vi "Autonics_1Scan_KAERI_lab2_Daejeon.vi"() -> ()   [LabVIEW 2018]
uses:
  <vilib>/Platform/NI_3dgraph.lvlib
  <vilib>/Utility/file.llb/Write To Spreadsheet File (DBL).vi
  <vilib>/Analysis/Matrix/Datatypes/RealMatrix.ctl
  <vilib>/Analysis/Matrix/NI_Matrix.lvlib
  <resource>/objmgr/daqmx.rc
  <vilib>/Instr/_visa.llb/VISA Configure Serial Port (Instr).vi
  <vilib>/DAQmx/configure/trigger.llb/DAQmx Start Trigger (Digital Edge).vi
  <vilib>/DAQmx/read.llb/DAQmx Read (Analog 2D DBL NChan NSamp).vi
  <vilib>/DAQmx/configure/timing.llb/DAQmx Timing (Sample Clock).vi
  <vilib>/DAQmx/create/channels.llb/DAQmx Create Channel (AI-Voltage-Basic).vi
  <vilib>/Utility/file.llb/Read From Spreadsheet File (DBL).vi
  <vilib>/Analysis/3filter.llb/Filter Passband Type.ctl
  <vilib>/Analysis/NI_AALBase.lvlib
panel:
  in  "Y-min":dbl
  in  "Y-max":dbl
  in  "Trim Data":bool
  in  "X-min":dbl
  in  "X-max":dbl
  out "XY Graph":cluster{"Array Repaired":dbl[], dbl[]}(graph)
  in  "dY":bool
  in  "dX":bool
  in  "Repair Line Y":bool
  in  "Repair Line X":bool
  in  "Line X":dbl
  in  "Line Y":dbl
  in  "Scan Mode":bool
  in  "3D Surface Analysis":refnum<k7>(container)
  in  "Auto Scale ?":bool
  out "Cursor Z":dbl=1.0
  out "Cursor Y":dbl=1.0
  out "Cursor X":dbl=1.0
  in  "Area View":bool
  in  "Save Analysis":bool caption="Save Process"
  in  "Color Max":dbl=1.0 step=0.01
  in  "Color Min":dbl step=0.01
  out "Section View Y":dbl[](graph) caption="Section View"
  in  "ViewMode Analysis":i32(ring) items=["cwViewXYPlane", "cwViewXZPlane", "cwViewYZPlane", "cwViewUserDefined"]
  in  "Plot style Analysis":i32(ring)=5 items=["cwLine"=1, "cwPoint"=2, "cwLinePoint"=3, "cwHiddenLine"=4, "cwSurface"=5, "cwSurfaceLine"=6, "cwSurfaceNormal"=7, "cwContourLine"=8, "cwSurfaceContour"=9]
  in  "Back data Analysis":bool
  in  "Direction":u16(ring) items=["X-dir", "Y-dir"]
  in  "Transpose ?":bool
  in  "filter type":T1
  in  "Filter?":bool
  in  "Order":dbl=2.0
  in  "Low Cutoff Hz":dbl=50.0
  in  "High Cutoff Hz":dbl=300.0
  in  "Sampling Hz":dbl=1000.0
  in  "Open":bool
  in  "Scan Distance":dbl=350.0
  in  "Save Button":bool caption="Save Process"
  in  "ViewMode":i32(ring) items=["cwViewXYPlane", "cwViewXZPlane", "cwViewYZPlane", "cwViewUserDefined"]
  in  "Back data":bool
  in  "Data Type":u16(ring) items=["Normal", "dX", "dY"]
  in  "Sampling Rate(Hz)":dbl=15000.0
  in  "Samples per Channels":i32=1000
  in  "Min Volts":dbl=-10.0 format="%0.2f"
  in  "Max Volts":dbl=10.0 format="%0.2f"
  in  "Channels":tag="Dev3/ai0:63"
  in  "Scan Step (mm)":dbl=1.0
  in  "Scan":bool
  in  "Plot style":i32(ring)=5 items=["cwLine"=1, "cwPoint"=2, "cwLinePoint"=3, "cwHiddenLine"=4, "cwSurface"=5, "cwSurfaceLine"=6, "cwSurfaceNormal"=7, "cwContourLine"=8, "cwSurfaceContour"=9]
  in  "3D Surface":refnum<k7>(container)
  in  "Flow control":u16(ring) items=["None", "XON/XOFF", "RTS/CTS", "XON/XOFF & RTS/CTS", "DTR/DSR", "XON/XOFF & DTR/DSR"]
  in  "Stop bits":u16(ring)=10 items=["1.0"=10, "1.5"=15, "2.0"=20]
  in  "Parity":dbl
  in  "Data bits":u16=8 min=5 max=8 step=1
  in  "Baud Rate":u32=57600
  in  "COM Port":refnum<visa-resource-name>="COM3"
  in  "Speed":dbl=10.0
  out "Current  Position (mm)":dbl format="%#_4g"
  in  "Move Distance (mm)":dbl=20.0
  in  "Stop Scan":bool
  in  "Stop":bool
  in  "Home":bool
  in  "Right":bool
  in  "Left":bool
  # "SCANNER CONTROL"
  # "BOBBIN-TYPE MAGNETIC CAMERA"
  # "CHANNELS"
  # "COM Setting"
  # "TIMING"
  # "DATA ANALYSIS"
  # "Filters"
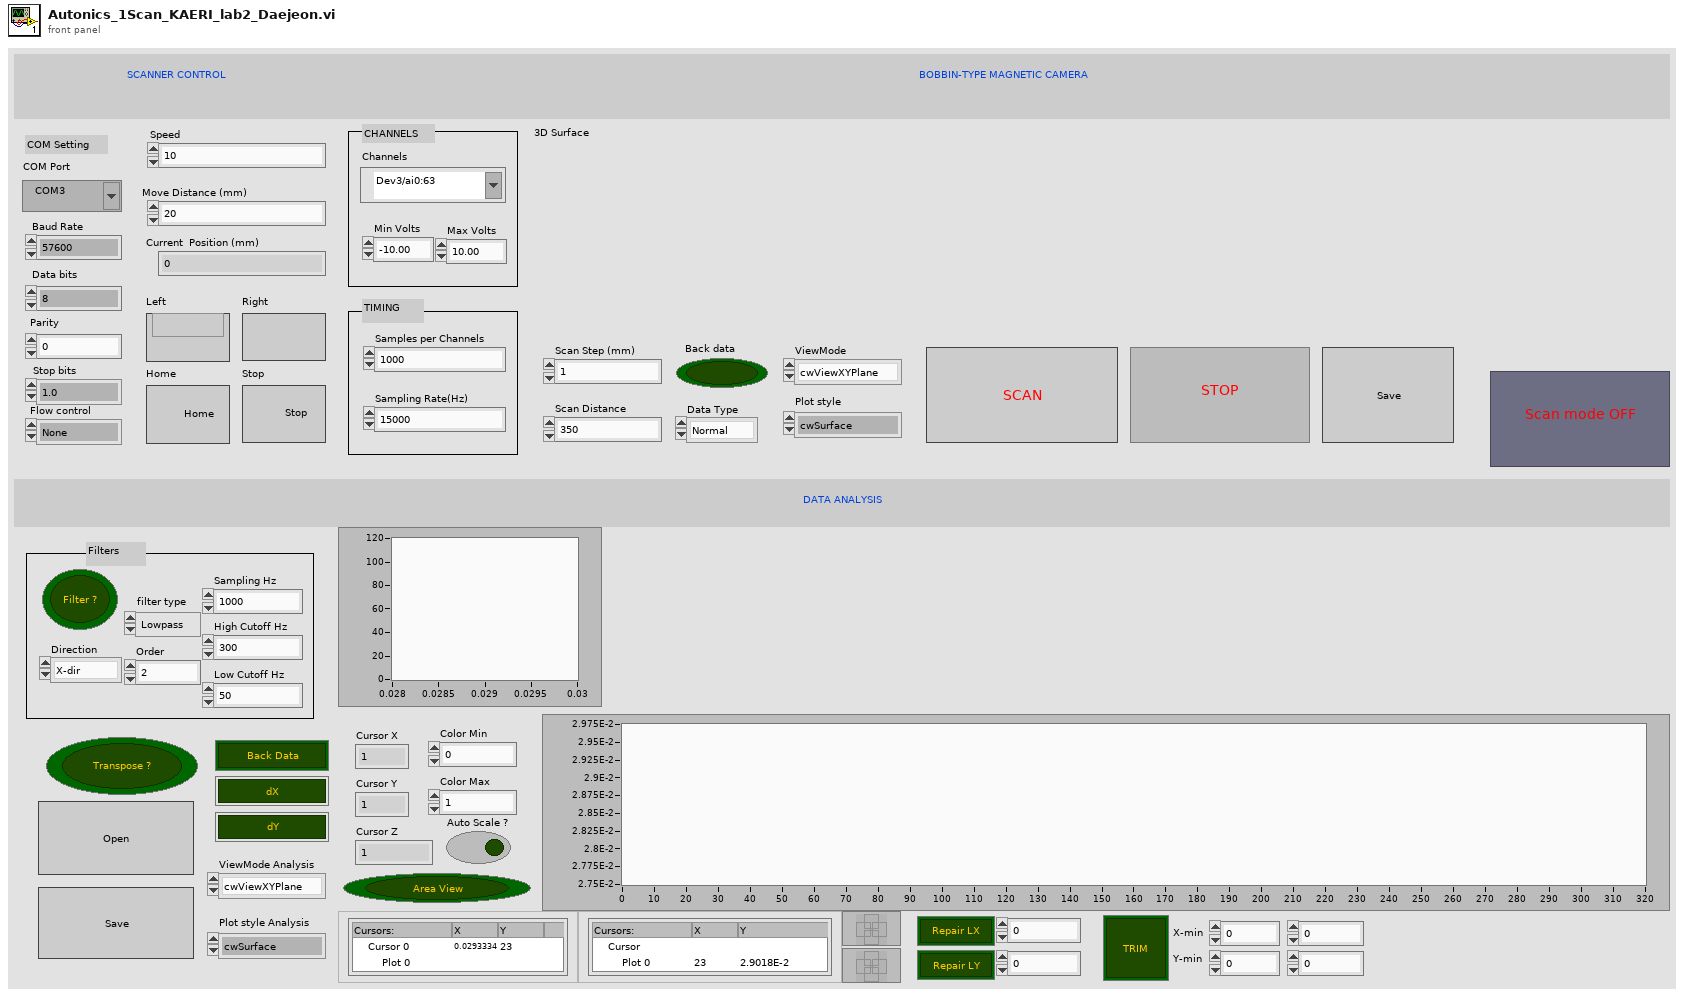
[diagram p1: front panel]
types:
  T1 = typedef "NI_AALBase.lvlib/Filter Passband Type.ctl" = enum32{"Lowpass", "Highpass", "Bandpass", "Bandstop"}
  T2 = typedef "NI_Matrix.lvlib/RealMatrix.ctl" = dbl[][]
  T3 = enum32{"Invalid", "Standard", "Closed", "Hidden", "Minimized", "Maximized"}
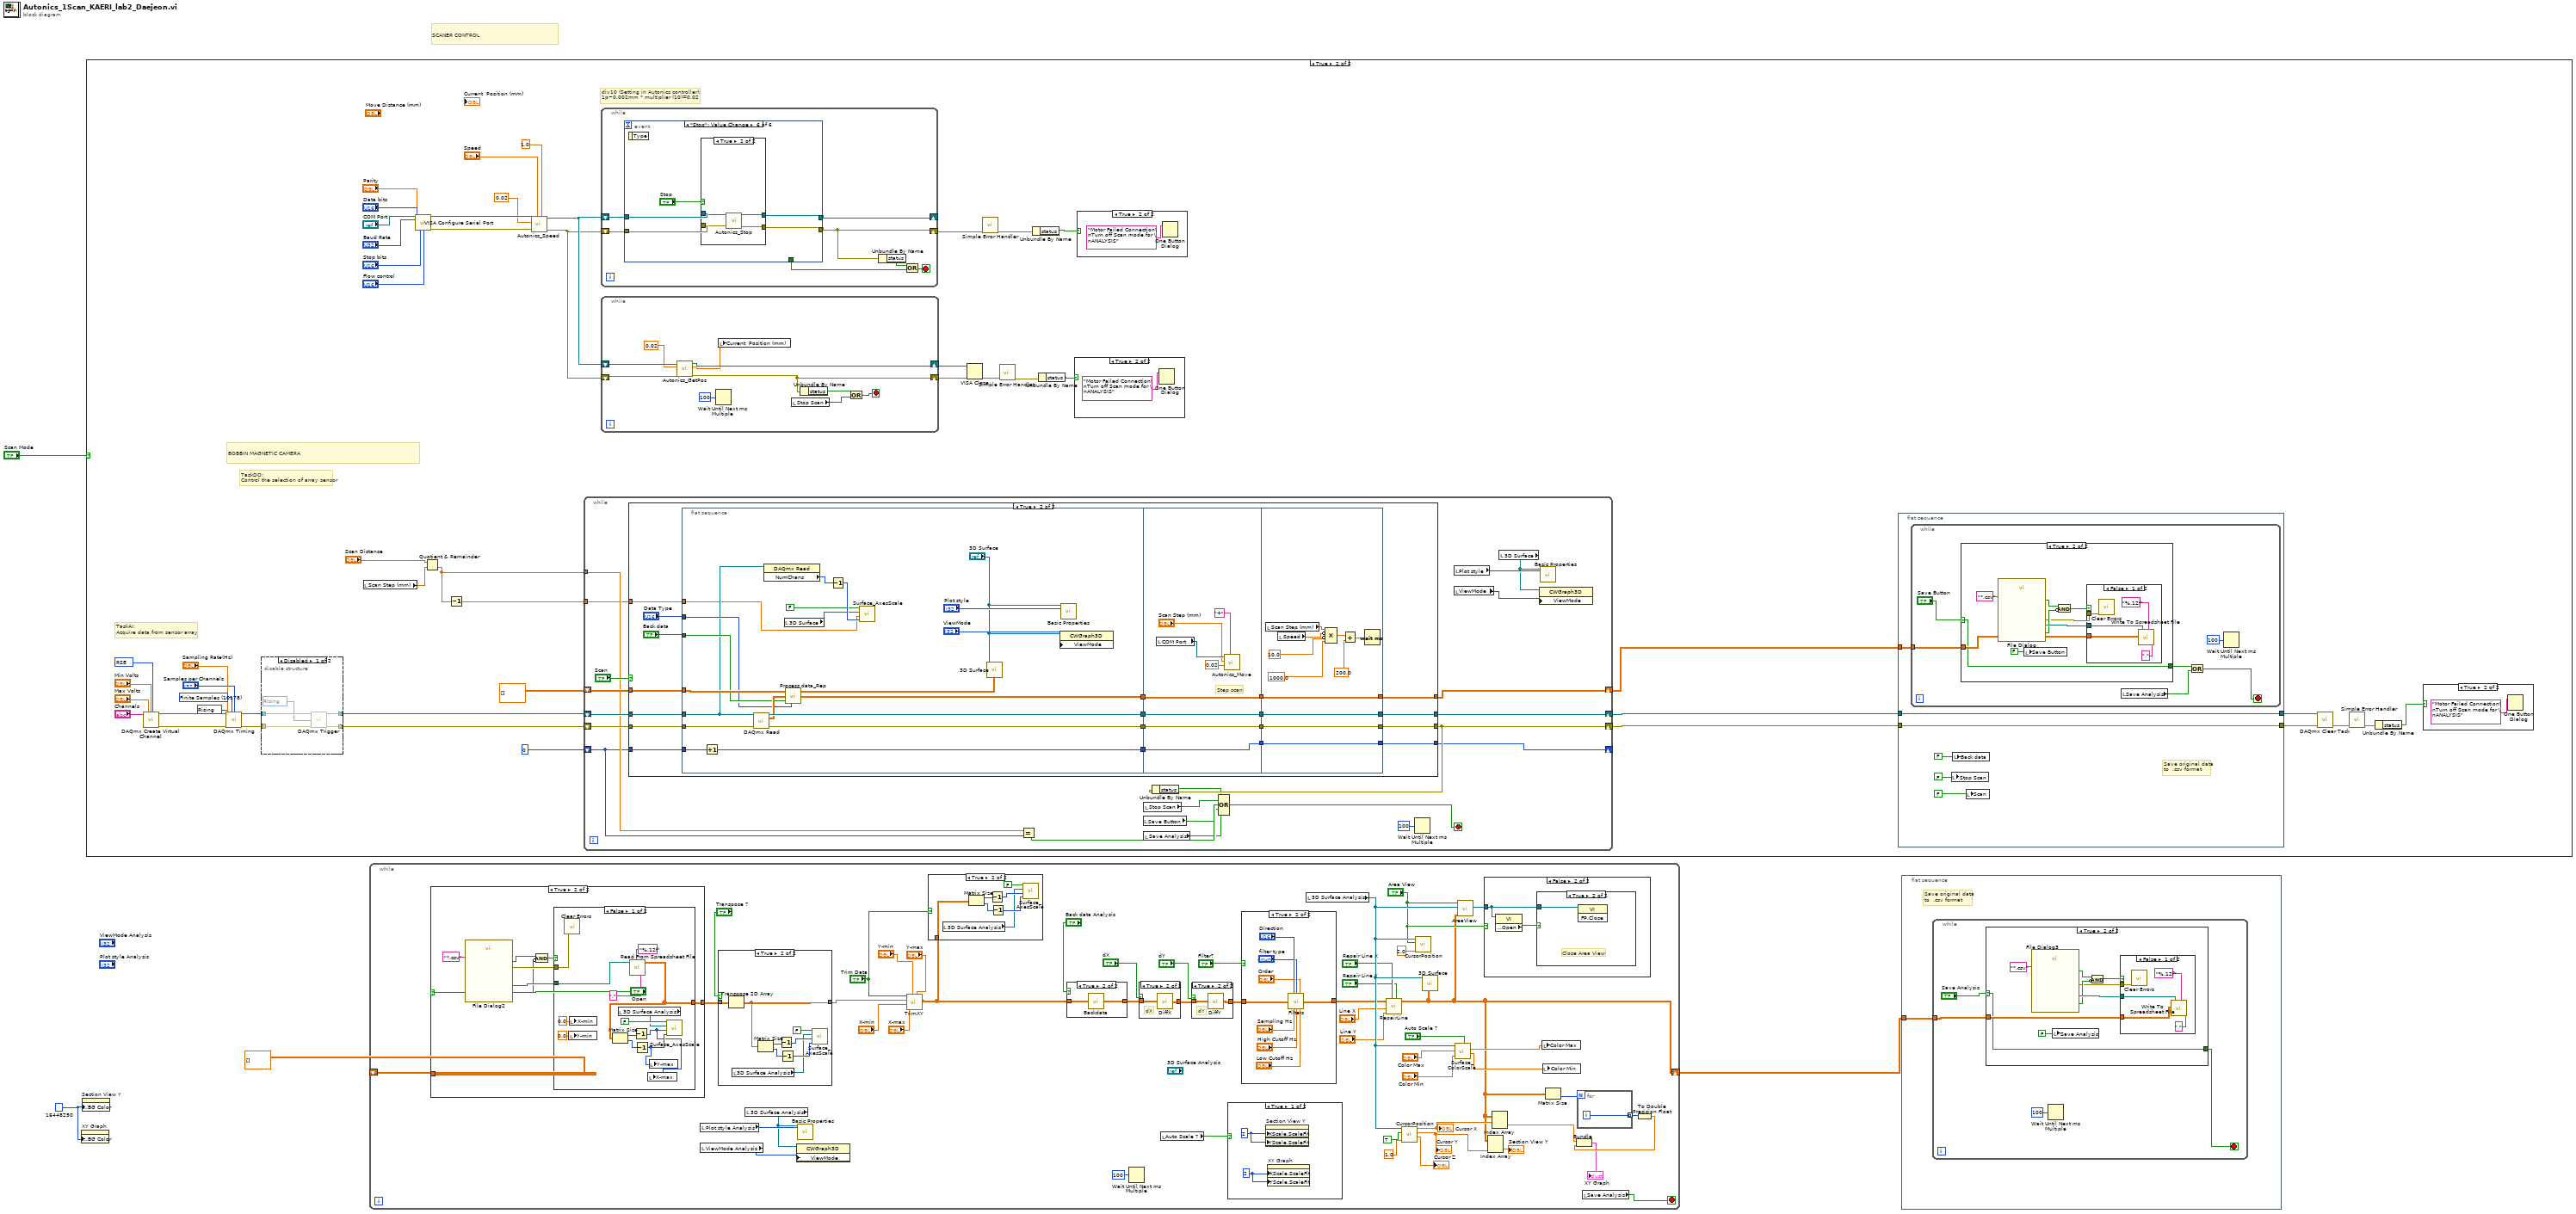
[diagram p0: block diagram]
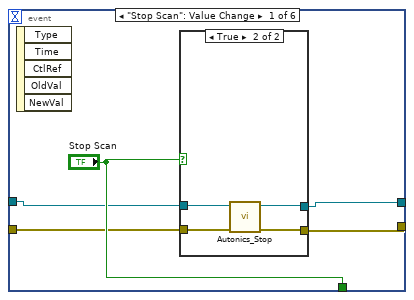
[diagram p6: hidden frame]
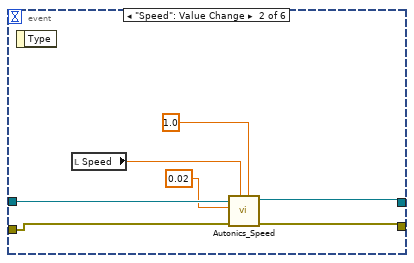
[diagram p8: hidden frame]
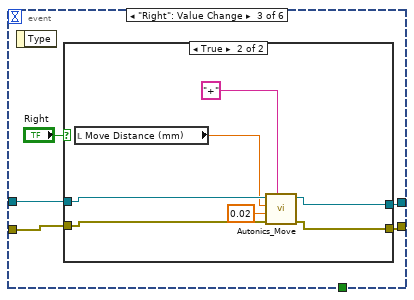
[diagram p9: hidden frame]
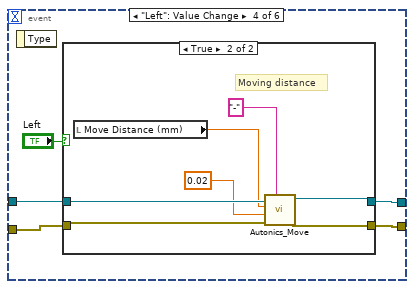
[diagram p11: hidden frame]
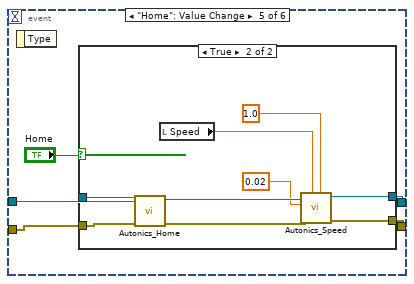
[diagram p13: hidden frame]
diagram:
  w1 = u32 16448250
  # "SCANER CONTROL"
  n1 = property on="XY Graph" class="XYGraph (strict)"("Plot Area:Colors:BG Color"=w1) -> ()  [unwired: 2 in, 2 out]
  n2 = property on="Section View Y" class="WFGraph (strict)"("Plot Area:Colors:BG Color"=w1) -> ()  [unwired: 2 in, 2 out]
  n3 = case shown="True" "Scan Mode" {
    frame False {
    }
    frame True {
      w36 = 10280 items=["Rising"=10280, "Falling"=10171] ("active edge")
      w45 = 10083 items=["default"=-1, "RSE"=10083, "NRSE"=10078, "Differential"=10106, "Pseudodifferential"=12529] ("input terminal configuration")
      w46 = 10178 items=["Finite Samples"=10178, "Continuous Samples"=10123, "Hardware Timed Single Point"=12522] ("sample mode")
      # "div10 (Setting in Autonics controller):\n1p~0.002mm * multiplier (10)=0.02"
      # "TaskAI:\nAcquire data from sensor array"
      # "TaskDO: \nControl the selection of array sensor"
      # "BOBBIN MAGNETIC CAMERA"
      n4 = call-poly <vilib>:"DAQmx Create Virtual Channel.vi"("maximum value"="Max Volts", "minimum value"="Min Volts", "input terminal configuration"=w45, "physical channels"="Channels") -> ("task out"=w53:refnum<k21>, "error out"=w52:errorcluster)  [unwired: 10 in]
      n5 = call-poly <vilib>:"DAQmx Timing.vi"("task/channels in"=w53, "sample mode"=w46, "samples per channel"="Samples per Channels", "rate"="Sampling Rate(Hz)", "active edge"=w36, "error in"=w52) -> ("task out"=w35:refnum<k21>, "error out"=w34:errorcluster)  [unwired: 8 in]
      n6 = disable-structure shown="Disabled" {
        disable-tunnel: w35 -> [w152 w154]
        disable-tunnel: [w151 w154] -> w30
        disable-tunnel: w34 -> [w150 w153]
        disable-tunnel: [w149 w153] -> w33
        frame Disabled {
          w148 = 10280 items=["Rising"=10280, "Falling"=10171] ("edge")
          n7 = call-poly <vilib>:"DAQmx Trigger.vi"("task/channels in"=w152, "edge"=w148, "error in"=w150) -> ("task out"=w151:refnum<k21>, "source"=w147:tag, "error out"=w149:errorcluster)  [unwired: 10 in]
        }
        frame Enabled {
        }
      }
      n8 = local read "Scan Step (mm)"() -> (w44:dbl)
      n9 = call-poly "VISA Configure Serial Port"("VISA resource name"="COM Port", "baud rate (9600)"="Baud Rate", "data bits (8)"="Data bits", "parity (0:none)"="Parity", "stop bits (10: 1 bit)"="Stop bits", "flow control (0:none)"="Flow control") -> ("VISA resource name out"=w16:refnum<visa-resource-name>, "error out"=w15:errorcluster)  [unwired: 8 in]
      n10 = Quotient & Remainder(x="Scan Distance", y=w44) -> (floor(x/y)=w32:dbl)  [unwired: 1 out]
      n11 = Decrement(x=w32) -> (x-1=w28:dbl)
      n12 = call "Autonics_Speed.vi"("Multiplier"=1.0, "Speed (mm/s)"="Speed", "error in (no error)"=w15, "Travel per  Pulse"=0.02, "VISA resource name"=w16) -> ("error out"=w18:errorcluster, "VISA resource name out"=w19:refnum<visa-resource-name>)  [unwired: 5 in]
      n13 = while {
        shift-right: [w185] -> w29
        shift-left: T2 [] ("Output (Matrix)") -> [w201]
        shift-right: [w199] -> w40
        shift-left: w30 -> [w200]
        shift-right: [w195] -> w38
        shift-left: w33 -> [w202]
        shift-right: [w193] -> _
        shift-left: 0 -> [w191]
        tunnel: w32 -> [w192]
        tunnel: w28 -> [w184]
        stop <- w198 stop-if-true
        n14 = case shown="True" "Scan" {
          tunnel: w200 -> [w205 w225]
          tunnel: w202 -> [w204 w224]
          tunnel: w201 -> [w203 w223]
          tunnel: [w205 w219] -> w199
          tunnel: [w204 w218] -> w195
          tunnel: [w203 w208] -> w185
          tunnel: [w206 w215] -> w193
          tunnel: w191 -> [w206 w213]
          tunnel: w184 -> [_ w207]
          frame False {
          }
          frame True {
            n15 = flat-sequence {
              tunnel: [w244] -> w222
              tunnel: [w235] -> w221
              tunnel: [w243] -> w220
              tunnel: [w234] -> w214
              tunnel: w225 -> [w227]
              tunnel: w224 -> [w245]
              tunnel: w223 -> [w239]
              tunnel: "Back data" -> [w237]
              tunnel: "Data Type" -> [w236]
              tunnel: w213 -> [w233]
              tunnel: w207 -> [w226]
              tunnel: w222 -> [w253]
              tunnel: w221 -> [w252]
              tunnel: w220 -> [w251]
              tunnel: w214 -> [w250]
              tunnel: [w253] -> w212
              tunnel: [w252] -> w211
              tunnel: [w251] -> w210
              tunnel: [w250] -> w209
              tunnel: [w261] -> w215
              tunnel: [w262] -> w218
              tunnel: [w263] -> w208
              tunnel: [w264] -> w219
              tunnel: w212 -> [w264]
              tunnel: w211 -> [w263]
              tunnel: w210 -> [w262]
              tunnel: w209 -> [w261]
              frame #0 {
                n16 = Increment(x=w233) -> (x+1=w234:i32)
                n17 = call-poly <vilib>:"DAQmx Read.vi"("task/channels in"=w227, "error in"=w245) -> ("task out"=w244:refnum<k21>, "data"=w238:dbl[][], "error out"=w243:errorcluster)  [unwired: 11 in]
                n18 = property class="DAQmx Read"(reference=w227) -> ("NumChans"=w230:u32)  [unwired: 1 in, 2 out]
                n19 = local read "3D Surface"() -> (w229:refnum<k7>)
                n20 = call "Process data_Rep.vi"("Initial Matrix"=w239, "Input Matrix"=w238, "Back Data"=w237, "Data Type"=w236) -> ("Process Output (Matrix)"=w232:T2, "Output (Matrix)"=w235:T2)  [unwired: 2 in]
                n21 = Decrement(x=w230) -> (x-1=w231:u32)
                n22 = call "Surface_AxesScale.vi"("Y-axis Max"=w231, "X-axis max"=w226, "3D Surface"=w229, "Auto Scale"=FALSE) -> ()  [unwired: 8 in]
                n23 = call <vilib>:"3D Surface.vi"("z matrix"=w232, "3D graph"="3D Surface") -> ()  [unwired: 8 in, 2 out]
                n24 = property class="CWGraph3D"(reference="3D Surface", "ViewMode"="ViewMode") -> ()  [unwired: 1 in, 2 out]
                n25 = call <vilib>:"Basic Properties.vi"("3D graph"="3D Surface", "plot style"="Plot style") -> ()  [unwired: 12 in, 2 out]
              }
              frame #1 {
                # "Step scan"
                n26 = local read "COM Port"() -> (w249:refnum<visa-resource-name>)
                n27 = call "Autonics_Move.vi"("Direction (+)"="+", "Travel per Pulse (mm)"=0.02, "Move Distance (mm)"="Scan Step (mm)", "VISA resource name"=w249) -> ()  [unwired: 6 in, 2 out]
              }
              frame #2 {
                n28 = local read "Scan Step (mm)"() -> (w256:dbl)
                n29 = local read "Speed"() -> (w257:dbl)
                n30 = Compound Arithmetic op=MULTIPLY(w256, invert w257, invert 10.0 ("value"), 1000.0 ("value")) -> (w258:dbl)
                n31 = Add(x=w258, y=200.0) -> (x+y=w260:dbl)
                n32 = Wait (ms)(milliseconds to wait=w260) -> ()  [unwired: 1 out]
              }
            }
          }
        }
        n33 = Equal?(x=w192, y=w191) -> (x = y?=w190:bool)
        n34 = local read "Save Button"() -> (w183:bool)
        n35 = local read "Stop Scan"() -> (w196:bool)
        n36 = local read "Save Analysis"() -> (w182:bool)
        n37 = Unbundle By Name(w195) -> ("status"=w194:bool)
        n38 = Compound Arithmetic op=OR(w194, w196, w190, w183, w182) -> (w198:bool)
        n39 = Wait Until Next ms Multiple(millisecond multiple=u32 100) -> ()  [unwired: 1 out]
        n40 = local read "Plot style"() -> (w188:i32)
        n41 = local read "ViewMode"() -> (w187:i32)
        n42 = local read "3D Surface"() -> (w186:refnum<k7>)
        n43 = property class="CWGraph3D"(reference=w186, "ViewMode"=w187) -> ()  [unwired: 1 in, 2 out]
        n44 = call <vilib>:"Basic Properties.vi"("3D graph"=w186, "plot style"=w188) -> ()  [unwired: 12 in, 2 out]
      }
      n45 = while {
        shift-right: [w73] -> _
        shift-left: w19 -> [w72]
        shift-right: [w69] -> w10
        shift-left: w18 -> [w71]
        stop <- w68 stop-if-true
        n46 = event shown="[5] \"Stop\": Value Change" {
          selector: _ -> [_ _ _ _ _ _]
          dyn-events: _ -> [_ _ _ _ _ _]
          timeout: _ -> [_ _ _ _ _ _]
          tunnel: w72 -> [w77 w91 w94 w108 w124 w138]
          tunnel: w71 -> [w76 w90 w93 w107 w123 w137]
          tunnel: [w75 w87 w96 w110 w121 w140] -> w73
          tunnel: [w74 w88 w95 w109 w120 w139] -> w69
          tunnel: ["Stop Scan" _ _ _ _ _] -> w67
          event "Stop Scan": Value Change {
            n47 = event-data() -> ()  [unwired: 1 in, 5 out]
            n48 = case shown="True" "Stop Scan" {
              tunnel: [w80 w83] -> w75
              tunnel: [w79 w84] -> w74
              tunnel: w77 -> [w80 w82]
              tunnel: w76 -> [w79 w81]
              frame False {
              }
              frame True {
                n49 = call "Autonics_Stop.vi"("error in (no error)"=w81, "VISA resource name"=w82) -> ("error out"=w84:errorcluster, "VISA resource name out"=w83:refnum<visa-resource-name>)  [unwired: 8 in]
              }
            }
          }
          event "Speed": Value Change {
            n50 = event-data() -> ()  [unwired: 1 in, 1 out]
            n51 = local read "Speed"() -> (w89:dbl)
            n52 = call "Autonics_Speed.vi"("Multiplier"=1.0, "Speed (mm/s)"=w89, "error in (no error)"=w90, "Travel per  Pulse"=0.02, "VISA resource name"=w91) -> ("error out"=w88:errorcluster, "VISA resource name out"=w87:refnum<visa-resource-name>)  [unwired: 5 in]
          }
          event "Right": Value Change {
            n53 = event-data() -> ()  [unwired: 1 in, 1 out]
            n54 = case shown="True" "Right" {
              tunnel: [w97 w103] -> w96
              tunnel: [w98 w102] -> w95
              tunnel: w94 -> [w97 w105]
              tunnel: w93 -> [w98 w104]
              frame False {
              }
              frame True {
                n55 = local read "Move Distance (mm)"() -> (w101:dbl)
                n56 = call "Autonics_Move.vi"("Direction (+)"="+", "error in (no error)"=w104, "Travel per Pulse (mm)"=0.02, "Move Distance (mm)"=w101, "VISA resource name"=w105) -> ("error out"=w102:errorcluster, "VISA resource name out"=w103:refnum<visa-resource-name>)  [unwired: 5 in]
              }
            }
          }
          event "Left": Value Change {
            n57 = event-data() -> ()  [unwired: 1 in, 1 out]
            n58 = case shown="True" "Left" {
              tunnel: [w112 w117] -> w110
              tunnel: [w111 w116] -> w109
              tunnel: w108 -> [w112 w119]
              tunnel: w107 -> [w111 w118]
              frame False {
              }
              frame True {
                # "Moving distance"
                n59 = local read "Move Distance (mm)"() -> (w114:dbl)
                n60 = call "Autonics_Move.vi"("Direction (+)"="-", "error in (no error)"=w118, "Travel per Pulse (mm)"=0.02, "Move Distance (mm)"=w114, "VISA resource name"=w119) -> ("error out"=w116:errorcluster, "VISA resource name out"=w117:refnum<visa-resource-name>)  [unwired: 5 in]
              }
            }
          }
          event "Home": Value Change {
            n61 = event-data() -> ()  [unwired: 1 in, 1 out]
            n62 = case shown="True" "Home" {
              tunnel: [w126 w130] -> w121
              tunnel: [w125 w129] -> w120
              tunnel: w124 -> [w126 w135]
              tunnel: w123 -> [w125 w134]
              frame False {
              }
              frame True {
                n63 = call "Autonics_Home.vi"("error in (no error)"=w134, "VISA resource name"=w135) -> ("error out"=w131:errorcluster, "VISA resource name out"=w132:refnum<visa-resource-name>)  [unwired: 8 in]
                n64 = local read "Speed"() -> (w133:dbl)
                n65 = call "Autonics_Speed.vi"("Multiplier"=1.0, "Speed (mm/s)"=w133, "error in (no error)"=w131, "Travel per  Pulse"=0.02, "VISA resource name"=w132) -> ("error out"=w129:errorcluster, "VISA resource name out"=w130:refnum<visa-resource-name>)  [unwired: 5 in]
              }
            }
          }
          event "Stop": Value Change {
            n66 = event-data() -> ()  [unwired: 1 in, 1 out]
            n67 = case shown="True" "Stop" {
              tunnel: [w142 w143] -> w140
              tunnel: [w141 w146] -> w139
              tunnel: w138 -> [w142 w145]
              tunnel: w137 -> [w141 w144]
              frame False {
              }
              frame True {
                n68 = call "Autonics_Stop.vi"("error in (no error)"=w144, "VISA resource name"=w145) -> ("error out"=w146:errorcluster, "VISA resource name out"=w143:refnum<visa-resource-name>)  [unwired: 8 in]
              }
            }
          }
        }
        n69 = Unbundle By Name(w69) -> ("status"=w70:bool)
        n70 = Compound Arithmetic op=OR(w70, w67) -> (w68:bool)
      }
      n71 = while {
        shift-right: [w61] -> w21
        shift-left: w19 -> [w63]
        shift-right: [w60] -> w20
        shift-left: w18 -> [w62]
        stop <- w64 stop-if-true
        n72 = call "Autonics_GetPos.vi"("error in (no error)"=w62, "Travel per Pulse (mm)"=0.02, "VISA resource name"=w63) -> ("error out"=w60:errorcluster, "Current  Position (mm)"=w59:dbl, "VISA resource name out"=w61:refnum<visa-resource-name>)  [unwired: 6 in]
        n73 = Wait Until Next ms Multiple(millisecond multiple=u32 100) -> ()  [unwired: 1 out]
        n74 = local write "Current  Position (mm)"(w59) -> ()
        n75 = local read "Stop Scan"() -> (w65:bool)
        n76 = Unbundle By Name(w60) -> ("status"=w57:bool)
        n77 = Compound Arithmetic op=OR(w57, w65) -> (w64:bool)
      }
      n78 = VISA Close(VISA resource name=w21, error in (no error)=w20) -> (error out=w8:errorcluster)
      n79 = call <vilib>:"Simple Error Handler.vi"("error in (no error)"=w10) -> ("error out"=w9:errorcluster)  [unwired: 4 in, 4 out]
      n80 = call <vilib>:"Simple Error Handler.vi"("error in (no error)"=w8) -> ("error out"=w7:errorcluster)  [unwired: 4 in, 4 out]
      n81 = Unbundle By Name(w9) -> ("status"=w12:bool)
      n82 = Unbundle By Name(w7) -> ("status"=w11:bool)
      n83 = case shown="True" w11 {
        frame False {
        }
        frame True {
          n84 = One Button Dialog(message="Motor Failed Connection\nTurn off Scan mode for \nANALYSIS") -> ()  [unwired: 1 in, 1 out]
        }
      }
      n85 = case shown="True" w12 {
        frame False {
        }
        frame True {
          n86 = One Button Dialog(message="Motor Failed Connection\nTurn off Scan mode for \nANALYSIS") -> ()  [unwired: 1 in, 1 out]
        }
      }
      n87 = flat-sequence {
        tunnel: w40 -> [w160]
        tunnel: [w160] -> w39
        tunnel: w38 -> [w159]
        tunnel: [w159] -> w37
        tunnel: w29 -> [w155]
        frame #0 {
          # "Save original data\nto  .csv format"
          n88 = while {
            tunnel: w155 -> [w166]
            stop <- w161 stop-if-true
            n89 = case shown="True" "Save Button" {
              selector: "Save Button" -> [w167 w169]
              tunnel: w166 -> [_ w176]
              tunnel: [w167 w169] -> w163
              frame False {
              }
              frame True {
                n90 = call "File Dialog"("pattern (all files)"="*.csv") -> ("selected path"=w174:path, "exists"=w172:bool, "cancelled"=w173:bool, "error out"=w170:errorcluster)  [unwired: 11 in]
                n91 = local write "Save Button"(FALSE ("Save Button")) -> ()
                n92 = Compound Arithmetic op=AND(w173, invert w172) -> (w171:bool)
                n93 = case shown="False" w171 {
                  tunnel: w176 -> [w181 _]
                  tunnel: w174 -> [w179 _]
                  tunnel: w170 -> [w177 _]
                  frame False {
                    n94 = call <vilib>:"Clear Errors.vi"("error in (no error)"=w177) -> ()  [unwired: 5 in, 2 out]
                    n95 = call-poly <vilib>:"Write To Spreadsheet File.vi"("delimiter (\\t)"="," ("delimiter (\\t)"), "format (%.3f)"="%.12f", "2D data"=w181, "file path (dialog if empty)"=w179) -> ()  [unwired: 4 in, 1 out]
                  }
                  frame True {
                  }
                }
              }
            }
            n96 = local read "Save Analysis"() -> (w162:bool)
            n97 = Compound Arithmetic op=OR(w163, w162) -> (w161:bool)
            n98 = Wait Until Next ms Multiple(millisecond multiple=u32 100) -> ()  [unwired: 1 out]
          }
          n99 = local write "Stop Scan"(FALSE ("Exit")) -> ()
          n100 = local write "Back data"(FALSE ("Back data")) -> ()
          n101 = local write "Scan"(FALSE ("Scan")) -> ()
        }
      }
      n102 = call <vilib>:"DAQmx Clear Task.vi"("task in"=w39, "error in"=w37) -> ("error out"=w41:errorcluster)  [unwired: 13 in]
      n103 = call <vilib>:"Simple Error Handler.vi"("error in (no error)"=w41) -> ("error out"=w6:errorcluster)  [unwired: 4 in, 4 out]
      n104 = Unbundle By Name(w6) -> ("status"=w5:bool)
      n105 = case shown="True" w5 {
        frame False {
        }
        frame True {
          n106 = One Button Dialog(message="Motor Failed Connection\nTurn off Scan mode for \nANALYSIS") -> ()  [unwired: 1 in, 1 out]
        }
      }
    }
  }
  n107 = while {
    shift-right: [w278] -> w2
    shift-left: T2 [] ("Output (Matrix)") -> [w314]
    stop <- w309 stop-if-true
    n108 = case shown="True" "Open" {
      tunnel: w314 -> [w339 _]
      tunnel: [w339 w346] -> w305
      frame False {
      }
      frame True {
        n109 = call "File Dialog2"("pattern (all files)"="*.csv") -> ("selected path"=w345:path, "exists"=w340:bool, "cancelled"=w341:bool, "error out"=w343:errorcluster)  [unwired: 11 in]
        n110 = Compound Arithmetic op=AND(w341, invert w340) -> (w342:bool)
        n111 = case shown="False" w342 {
          tunnel: w345 -> [w359 _]
          tunnel: [w358 _] -> w346
          tunnel: w343 -> [w357 _]
          frame False {
            n112 = call <vilib>:"Clear Errors.vi"("error in (no error)"=w357) -> ()  [unwired: 5 in, 2 out]
            n113 = local write "Y-min"(0.0 ("Y-min")) -> ()
            n114 = local write "X-min"(0.0 ("X-min")) -> ()
            n115 = local read "3D Surface Analysis"() -> (w351:refnum<k7>)
            n116 = call-poly <vilib>:"Read From Spreadsheet File.vi"("delimiter (\\t)"="," ("delimiter (\\t)"), "format (%.3f)"="%.12f", "file path (dialog if empty)"=w359) -> ("all rows"=w358:dbl[][])  [unwired: 4 in, 4 out]
            n117 = Matrix Size(0:w358) -> (1:w354:i32, 2:w353:i32)
            n118 = Decrement(x=w354) -> (x-1=w347:i32)
            n119 = Decrement(x=w353) -> (x-1=w348:i32)
            n120 = local write "X-max"(w347) -> ()
            n121 = local write "Y-max"(w348) -> ()
            n122 = call "Surface_AxesScale.vi"("Y-axis Max"=w348, "X-axis max"=w347, "3D Surface"=w351, "Auto Scale"=FALSE) -> ()  [unwired: 8 in]
          }
          frame True {
          }
        }
      }
    }
    n123 = local read "Plot style Analysis"() -> (w308:i32)
    n124 = local read "ViewMode Analysis"() -> (w307:i32)
    n125 = case shown="True" "Transpose ?" {
      tunnel: w305 -> [w360 w368]
      tunnel: [w360 w362] -> w272
      frame False {
      }
      frame True {
        n126 = Transpose 2D Array(2D array=w368) -> (transposed array=w362:T2)
        n127 = local read "3D Surface Analysis"() -> (w361:refnum<k7>)
        n128 = Matrix Size(0:w362) -> (1:w363:i32, 2:w364:i32)
        n129 = Decrement(x=w363) -> (x-1=w366:i32)
        n130 = Decrement(x=w364) -> (x-1=w367:i32)
        n131 = call "Surface_AxesScale.vi"("Y-axis Max"=w367, "X-axis max"=w366, "3D Surface"=w361, "Auto Scale"=FALSE) -> ()  [unwired: 8 in]
      }
    }
    n132 = local read "3D Surface Analysis"() -> (w306:refnum<k7>)
    n133 = property class="CWGraph3D"(reference=w306, "ViewMode"=w307) -> ()  [unwired: 1 in, 2 out]
    n134 = call <vilib>:"Basic Properties.vi"("3D graph"=w306, "plot style"=w308) -> ()  [unwired: 12 in, 2 out]
    n135 = call "TrimXY.vi"("X-max"="Y-max", "X-min"="Y-min", "Y-max"="X-max", "Y-min"="X-min", "Array In"=w272, "Trim data"="Trim Data") -> ("Array Trim Out"=w265:dbl[][])  [unwired: 5 in]
    n136 = case shown="True" "Trim Data" {
      tunnel: w265 -> [_ w315]
      frame False {
      }
      frame True {
        n137 = local read "3D Surface Analysis"() -> (w316:refnum<k7>)
        n138 = Matrix Size(0:w315) -> (1:w317:i32, 2:w318:i32)
        n139 = Decrement(x=w317) -> (x-1=w320:i32)
        n140 = Decrement(x=w318) -> (x-1=w321:i32)
        n141 = call "Surface_AxesScale.vi"("Y-axis Max"=w321, "X-axis max"=w320, "3D Surface"=w316, "Auto Scale"=FALSE) -> ()  [unwired: 8 in]
      }
    }
    n142 = case shown="True" "Back data Analysis" {
      tunnel: w265 -> [w378 w379]
      tunnel: [w378 w380] -> w289
      frame False {
      }
      frame True {
        n143 = call "Backdata.vi"("Input Matrix"=w379) -> ("Backdata (matrix)"=w380:T2)
      }
    }
    n144 = Wait Until Next ms Multiple(millisecond multiple=u32 100) -> ()  [unwired: 1 out]
    n145 = case shown="True" "dX" {
      tunnel: [w330 w332] -> w287
      tunnel: w289 -> [w330 w331]
      frame False {
      }
      frame True {
        # "dX"
        n146 = call "DiffX.vi"("Input Matrix"=w331) -> ("Diff X (Matrix)"=w332:T2)
      }
    }
    n147 = local read "Auto Scale ?"() -> (w267:bool)
    n148 = case shown="True" "dY" {
      tunnel: w287 -> [w327 w328]
      tunnel: [w327 w329] -> w285
      frame False {
      }
      frame True {
        # "dY"
        n149 = call "DiffY.vi"("Input Matrix"=w328) -> ("Diff Y (Matrix)"=w329:T2)
      }
    }
    n150 = case shown="True" w267 {
      frame True {
        w322 = u8 2 ("X Scale.Scale Fit")
        w323 = u8 2 ("X Scale.Scale Fit")
        n151 = property on="Section View Y" class="WFGraph (strict)"("XScale.ScaleFit"=w323, "YScale.ScaleFit"=w323) -> ()  [unwired: 2 in, 2 out]
        n152 = property on="XY Graph" class="XYGraph (strict)"("XScale.ScaleFit"=w322, "YScale.ScaleFit"=w322) -> ()  [unwired: 2 in, 2 out]
      }
      frame False {
        w324 = u8 0 ("X Scale.Scale Fit")
        w325 = u8 0 ("X Scale.Scale Fit")
        n153 = property on="XY Graph" class="XYGraph (strict)"("XScale.ScaleFit"=w324, "YScale.ScaleFit"=w324) -> ()  [unwired: 2 in, 2 out]
        n154 = property on="Section View Y" class="WFGraph (strict)"("XScale.ScaleFit"=w325, "YScale.ScaleFit"=w325) -> ()  [unwired: 2 in, 2 out]
      }
    }
    n155 = case shown="True" "Filter?" {
      tunnel: [w369 w371] -> w284
      tunnel: w285 -> [w369 w370]
      frame False {
      }
      frame True {
        n156 = call "Filters.vi"("Direction"="Direction", "filter type"="filter type", "Order"="Order", "Input data"=w370, "Sampling Freq"="Sampling Hz", "High Cutoff Freq"="High Cutoff Hz", "Low Cutoff Freq"="Low Cutoff Hz") -> ("Filterd Data Matrix"=w371:T2)  [unwired: 8 in]
      }
    }
    n157 = local read "3D Surface Analysis"() -> (w304:refnum<k7>)
    n158 = call "RepairLine.vi"("Repair Line Col"="Repair Line Y", "Repair Line Row"="Repair Line X", "Line Col"="Line Y", "Line Row"="Line X", "Array In"=w284) -> ("Array Repaired"=w278:dbl[][])  [unwired: 6 in]
    n159 = call "CursorPosition.vi"("Cursor No."=1.0, "Cursor"=TRUE ("Visible"), "3D Surface Analysis"=w304) -> ("Cursor Z"=→"Cursor Z":dbl, "Cursor Y"=w295:dbl, "Cursor X"=w279:dbl)  [unwired: 6 in]
    "Cursor X" <- w279
    "Cursor Y" <- w295
    n160 = call "CursorPosition.vi"("Cursor No."=2.0, "Cursor"="Area View", "3D Surface Analysis"=w304) -> ()  [unwired: 6 in, 3 out]
    n161 = call <vilib>:"3D Surface.vi"("z matrix"=w278, "3D graph"=w304) -> ()  [unwired: 8 in, 2 out]
    n162 = call "Surface_ColorScale.vi"("ColorMapAutoScale"="Auto Scale ?", "Min"="Color Min", "Max"="Color Max", "3D Surface_"=w304) -> ("Min 2"=w299:dbl, "Max 2"=w300:dbl)  [unwired: 1 in, 2 out]
    n163 = call "AreaView.vi"("Real Matrix"=w278, "3D Surface Analysis"=w304, "Area View"="Area View") -> ("This VI"=w297:refnum<vi>)  [unwired: 7 in, 1 out]
    n164 = case shown="False" "Area View" {
      tunnel: w297 -> [w335 w337]
      frame True {
        # "Open Area View"
        n165 = invoke class="VI" method="FP.Open"(reference=w335, "Activate"=TRUE ("Activate?"), "State"=T3."Standard") -> ()  [unwired: 2 in, 5 out]
      }
      frame False {
        n166 = property class="VI"(reference=w337) -> ("Front Panel.Open"=w336:bool)  [unwired: 1 in, 2 out]
        n167 = case shown="True" w336 {
          tunnel: w337 -> [_ w338]
          frame False {
          }
          frame True {
            # "Close Area View"
            n168 = invoke class="VI" method="FP.Close"(reference=w338) -> ()  [unwired: 2 in, 3 out]
          }
        }
      }
    }
    n169 = Index Array(array=w278, index (col)=w295) -> (element=→"Section View Y":dbl[])  [unwired: 1 in]
    n170 = Index Array(array=w278, index (row)=w279) -> (element=w276:dbl[])  [unwired: 1 in]
    n171 = local write "Color Max"(w300) -> ()
    n172 = local write "Color Min"(w299) -> ()
    n173 = Matrix Size(0:w278) -> (2:w277:i32)  [unwired: 1 out]
    n174 = for {
      N: w277 -> [_]
      tunnel: [w326] -> w275 mode=indexing
      i -> [w326]
    }
    n175 = local read "Save Analysis"() -> (w309:bool)
    n176 = To Double Precision Float(number=w275) -> (double precision float=w274:dbl[])
    n177 = Bundle("Array Repaired"=w276, w274) -> (→"XY Graph":cluster{"Array Repaired":dbl[], dbl[]})  [unwired: 1 in]
  }
  n178 = flat-sequence {
    tunnel: w2 -> [w381]
    frame #0 {
      # "Save original data\nto  .csv format"
      n179 = while {
        tunnel: w381 -> [w385]
        stop <- w383 stop-if-true
        n180 = case shown="True" "Save Analysis" {
          selector: "Save Analysis" -> [w386 w388]
          tunnel: w385 -> [_ w389]
          tunnel: [w386 w388] -> w383
          frame False {
          }
          frame True {
            n181 = call "File Dialog3"("pattern (all files)"="*.csv") -> ("selected path"=w394:path, "exists"=w392:bool, "cancelled"=w393:bool, "error out"=w390:errorcluster)  [unwired: 11 in]
            n182 = local write "Save Analysis"(FALSE ("Save Analysis")) -> ()
            n183 = Compound Arithmetic op=AND(w393, invert w392) -> (w391:bool)
            n184 = case shown="False" w391 {
              tunnel: w394 -> [w399 _]
              tunnel: w390 -> [w397 _]
              tunnel: w389 -> [w396 _]
              frame False {
                n185 = call <vilib>:"Clear Errors.vi"("error in (no error)"=w397) -> ()  [unwired: 5 in, 2 out]
                n186 = call-poly <vilib>:"Write To Spreadsheet File.vi"("delimiter (\\t)"="," ("delimiter (\\t)"), "format (%.3f)"="%.12f", "2D data"=w396, "file path (dialog if empty)"=w399) -> ()  [unwired: 4 in, 1 out]
              }
              frame True {
              }
            }
          }
        }
        n187 = Wait Until Next ms Multiple(millisecond multiple=u32 100) -> ()  [unwired: 1 out]
      }
    }
  }
